vi "Audio read LV.vi"() -> ()   [LabVIEW 2025]
uses:
  <vilib>/sound2/lvsound2.llb/Sampling Mode.ctl
  <vilib>/sound2/lvsound2.llb/Sound Data Format.ctl
  <vilib>/sound2/lvsound2.llb/Sound File Refnum.ctl
  <vilib>/Analysis/2dsp.llb/Real FFT.vi
  <vilib>/sound2/lvsound2.llb/Sound Input Read (DBL).vi
  <vilib>/sound2/lvsound2.llb/Sound File Write (DBL).vi
  <vilib>/Analysis/NI_AALPro.lvlib
  <vilib>/sound2/lvsound2.llb/Sound File Write Open.vi
panel:
  in  "Stop\nRecord":bool
  in  "Save File in":path=path "D:/nagam/Documents/AudioWriteLV.wav"
  in  "Clear":bool
  in  "Start\nRecord":bool
  out "Spectrum Graph":dbl[](graph)
  in  "stop":bool
  out "Sound Output":waveform(dbl)[](graph)
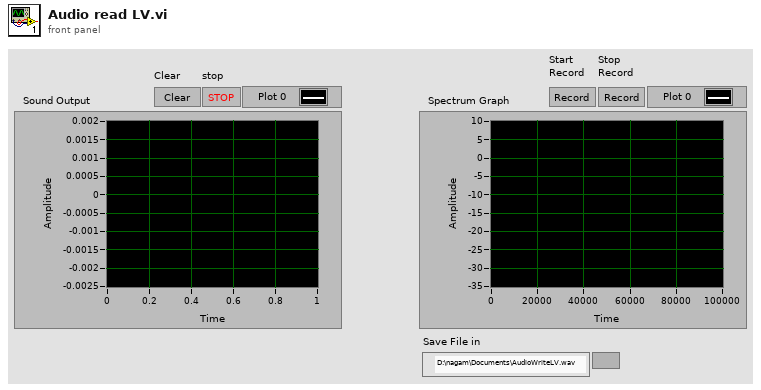
[diagram p1: front panel]
types:
  T1 = typedef "Sound Data Format.ctl" = cluster{"sample rate (S/s)":dbl, "number of channels":i32, "bits per sample":i32}
  T2 = typedef "Sampling Mode.ctl" = i32
  T3 = typedef "Sound Input Task ID.ctl" = u32
  T4 = typedef "Sound File Refnum.ctl" = refnum<file>
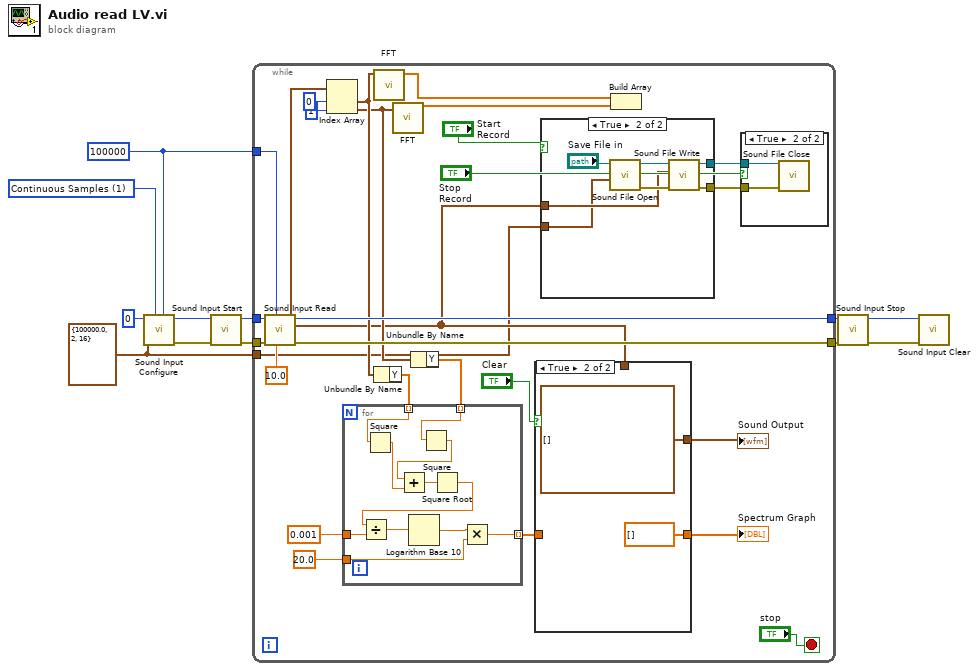
[diagram p0: block diagram]
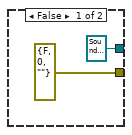
[diagram p4: hidden frame]
diagram:
  w1 = T1 {"sample rate (S/s)"=100000.0, "number of channels"=2, "bits per sample"=16} ("sound format")
  w12 = T2 1 items=["Finite Samples", "Continuous Samples"] ("sample mode")
  w2 = 100000 ("number of samples/ch")
  n1 = call <vilib>:"Sound Input Configure.vi"("number of samples/ch"=w2, "sample mode"=w12, "sound format"=w1, "device ID"=u32 0) -> ("error out"=w9:errorcluster, "task ID"=w10:T3)  [unwired: 6 in]
  n2 = call <vilib>:"Sound Input Start.vi"("error in (no error)"=w9, "task ID"=w10) -> ("error out"=w7:errorcluster, "task ID out"=w8:T3)  [unwired: 8 in]
  n3 = while {
    tunnel: w8 -> [w39]
    tunnel: w7 -> [w38]
    tunnel: [w36] -> w6
    tunnel: [w35] -> w5
    tunnel: w2 -> [w32]
    tunnel: w1 -> [w13]
    stop <- "stop" stop-if-true
    n4 = call-poly <vilib>:"Sound Input Read.vi"("timeout (sec)"=10.0, "number of samples/ch"=w32, "error in (no error)"=w38, "task ID"=w39) -> ("error out"=w35:errorcluster, "data"=w20:waveform(dbl)[], "task ID out"=w36:T3)  [unwired: 5 in]
    n5 = Index Array(array=w20, index #1=0 ("index"), index #2=1 ("index")) -> (element #1=w29:waveform(dbl), element #2=w28:waveform(dbl))
    n6 = call-poly <vilib>:"FFT.vi"("X"=w29) -> ("FFT {X}"=w31:cdb[])  [unwired: 9 in, 1 out]
    n7 = Unbundle By Name(w29) -> ("Y"=w27:dbl[])
    n8 = call-poly <vilib>:"FFT.vi"("X"=w28) -> ("FFT {X}"=w30:cdb[])  [unwired: 9 in, 1 out]
    n9 = Unbundle By Name(w28) -> ("Y"=w26:dbl[])
    n10 = for {
      tunnel: w27 -> [w64] mode=indexing
      tunnel: w26 -> [w63] mode=indexing
      tunnel: 0.001 ("y") -> [w59]
      tunnel: 20.0 ("y") -> [w56]
      tunnel: [w55] -> w18 mode=indexing
      n11 = Square(x=w64) -> (x^2=w61:dbl)
      n12 = Square(x=w63) -> (x^2=w62:dbl)
      n13 = Add(x=w62, y=w61) -> (x+y=w65:dbl)
      n14 = Square Root(x=w65) -> (sqrt(x)=w60:dbl)
      n15 = Divide(x=w60, y=w59) -> (x/y=w58:dbl)
      n16 = Logarithm Base 10(1:w58) -> (0:w57:dbl)
      n17 = Multiply(x=w57, y=w56) -> (x*y=w55:dbl)
    }
    n18 = case shown="True" "Clear" {
      tunnel: [w43 waveform(dbl)[] [] ("data")] -> w21
      tunnel: w20 -> [w43 _]
      tunnel: [w42 dbl[] []] -> w19
      tunnel: w18 -> [w42 _]
      frame False {
      }
      frame True {
      }
    }
    "Sound Output" <- w21
    "Spectrum Graph" <- w19
    n19 = case shown="True" "Start\nRecord" {
      tunnel: w20 -> [_ w52]
      tunnel: [errorcluster {"status"=FALSE, "code"=0, "source"=""} ("error out") w50] -> w17
      tunnel: [T4 refnum ("sound file refnum out") w49] -> w16
      tunnel: w13 -> [_ w48]
      frame False {
      }
      frame True {
        n20 = call-poly <vilib>:"Sound File Open.vi"("sound format"=w48, "path"="Save File in") -> ("error out"=w54:errorcluster, "sound file refnum"=w53:T4)  [unwired: 8 in]
        n21 = call-poly <vilib>:"Sound File Write.vi"("error in (no error)"=w54, "data"=w52, "sound file refnum"=w53) -> ("error out"=w50:errorcluster, "sound file refnum out"=w49:T4)  [unwired: 7 in]
      }
    }
    n22 = Build Array(w31, w30) -> ()  [unwired: 1 out]
    n23 = case shown="True" "Stop\nRecord" {
      tunnel: w17 -> [_ w41]
      tunnel: w16 -> [_ w40]
      frame False {
      }
      frame True {
        n24 = call <vilib>:"Sound File Close.vi"("error in (no error)"=w41, "sound file refnum"=w40) -> ()  [unwired: 9 in, 1 out]
      }
    }
  }
  n25 = call <vilib>:"Sound Input Stop.vi"("error in (no error)"=w5, "task ID"=w6) -> ("error out"=w3:errorcluster, "task ID out"=w4:T3)  [unwired: 8 in]
  n26 = call <vilib>:"Sound Input Clear.vi"("error in (no error)"=w3, "task ID"=w4) -> ()  [unwired: 9 in, 1 out]
